vi "CALC_DATA_SNP_S.vi"(0 "VISA IN":refnum<visa-resource-name>, 1 "Cmd 1":i32, 5 "error in":errorcluster, 7 "Channel":i32) -> (14 "VISA Out":refnum<visa-resource-name>, 16 "Data":string, 19 "error out":errorcluster)   [LabVIEW 2018, in "PNA-X.lvlib"]
doc: "CALCulate<cnum>:DATA:SNP? <n> Superseded \nNote: This command has been replaced by CALC:DATA:SNP:PORTs? \n(Read-only) Reads SnP data from the selected measurement. Learn more about SnP data. \nNote: This command returns SNP data without header information, and in columns, not in rows as \n.SnP files. This means that the data returned from this command sends all frequency data, then all Sx1 \nmagnitude data, then all Sx1 phase data, and so forth. \nSee Critical Note \nParameters \n<cnum> Channel number of the measurement. There must be a selected measurement \non that channel. If unspecified, <cnum> is set to 1. \n<n> Amount of data to return. If unspecified, <n> is set to 2. The number you \nspecify must be less than or equal to the number of available ports on the PNA. \nChoose from: \n1 (S1P) returns data for the active measurement. \n2 (S2P) returns data for the 2 port parameters associated with the current \nmeasurement. Default. \n3 (S3P) returns data for the 3 port parameters associated with the current \nmeasurement. \n4 (S4P) returns data for the 4 port parameters associated with the current \n1500\n\nmeasurement. \nSnP data can be output using several data formatting options. See \nMMEM:STORe:TRACe:FORMat:SNP. \nSee also MMEM:STOR <file>.<snp> \nExamples CALC:PAR:DEF �MyMeasurement�, S11 \nCALC:PAR:SEL �MyMeasurement� \nCALC:DATA:SNP? 1 \nReturn Type Depends on FORMat:DATA \nDefault Not Applicable"
uses:
  PNA-X.lvlib
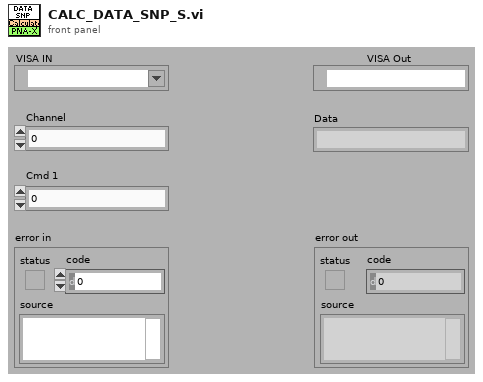
[diagram p1: front panel]
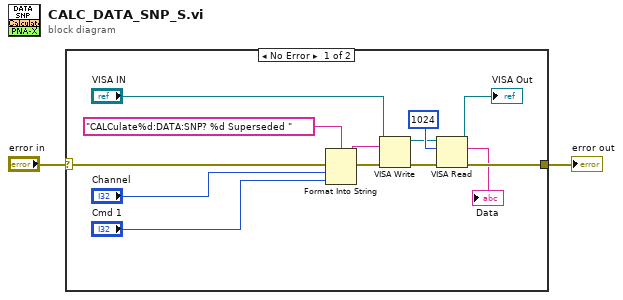
[diagram p0: block diagram]
diagram:
  n1 = case shown="No Error" "error in" {
    selector: "error in" -> [w15 w16]
    tunnel: [w7 w16] -> w1
    frame No Error {
      n2 = Format Into String(format string="CALCulate%d:DATA:SNP? %d Superseded " ("Cmdline"), error in=w15, "Channel", "Cmd 1") -> (resulting string=w13:string, error out=w14:errorcluster)  [unwired: 1 in]
      n3 = VISA Write(VISA resource name="VISA IN", write buffer=w13, error in (no error)=w14) -> (VISA resource name out=w8:refnum<visa-resource-name>, error out=w10:errorcluster)  [unwired: 1 out]
      n4 = VISA Read(VISA resource name=w8, byte count=1024, error in (no error)=w10) -> (VISA resource name out=→"VISA Out":refnum<visa-resource-name>, read buffer=→"Data":string, error out=w7:errorcluster)  [unwired: 1 out]
    }
    frame Error {
    }
  }
  "error out" <- w1
